vi "_PC_Pub_ExpCondi getAttributeValue.vi"(7 "attrName":string="Script", 8 "error in (no error)":errorcluster, 11 "expCondiVariant":variant) -> (0 "error out":errorcluster, 3 "attrValue":cluster{"Label":string, "Value":variant})   [LabVIEW 2018]
uses:
  <vilib>/Utility/error.llb/Error Cluster From Error Code.vi
  <vilib>/ErrorRing/Error Ring.xnode
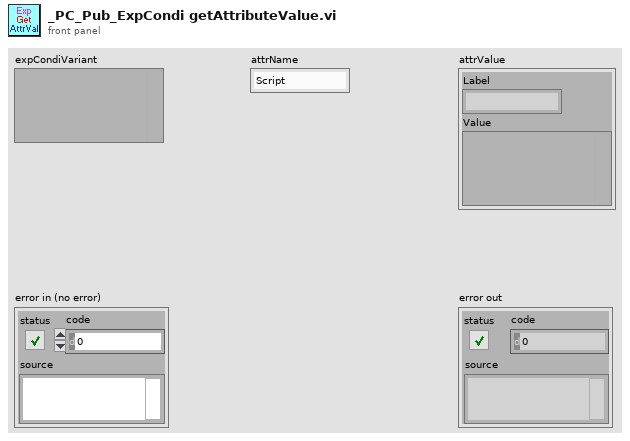
[diagram p1: front panel]
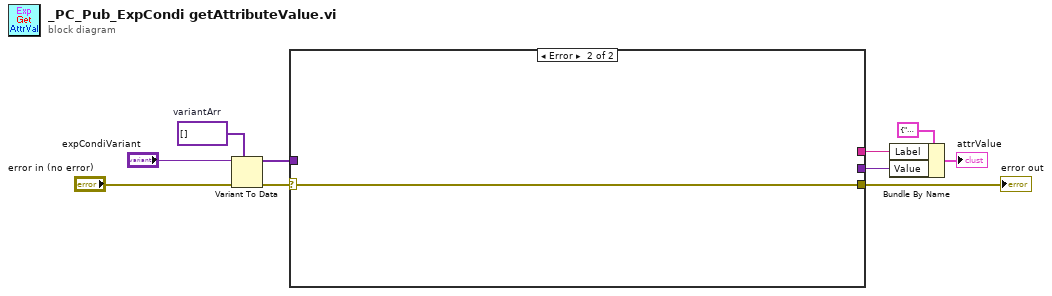
[diagram p0: block diagram]
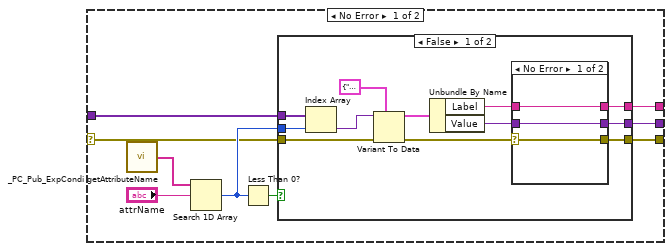
[diagram p2: hidden frame]
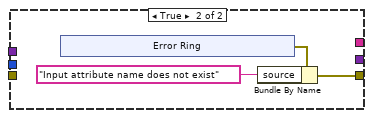
[diagram p4: hidden frame]
diagram:
  w8 = variant[] []  # variantArr
  n1 = Variant To Data(error in="error in (no error)", type=w8, Variant="expCondiVariant") -> (data=w7:variant[], error out=w6:errorcluster)
  n2 = case shown="Error" w6 {
    selector: w6 -> [w13 w43]
    tunnel: [w17 w43] -> w10
    tunnel: w7 -> [w16 _]
    tunnel: [w12 _] -> w4
    tunnel: [w11 _] -> w3
    frame No Error {
      n3 = call "_PC_Pub_ExpCondi getAttributeName.vi"() -> ("attrName"=w19:string[])
      n4 = Search 1D Array(1D array=w19, element="attrName") -> (index of element=w15:i32)  [unwired: 1 in]
      n5 = Less Than 0?(x=w15) -> (x < 0?=w18:bool)
      n6 = case shown="False" w18 {
        tunnel: [w24 w36] -> w17
        tunnel: w16 -> [w31 _]
        tunnel: w15 -> [w30 _]
        tunnel: w13 -> [w26 _]
        tunnel: [w21 _] -> w12
        tunnel: [w20 _] -> w11
        frame False {
          n7 = Index Array(array=w31, index=w30) -> (element=w29:variant)
          n8 = Variant To Data(error in=w26, type=cluster{"Label":string, "Value":variant} {"Label"="", "Value"=variant} ("element"), Variant=w29) -> (data=w27:cluster{"Label":string, "Value":variant}, error out=w25:errorcluster)
          n9 = Unbundle By Name(w27) -> ("Label"=w23:string, "Value"=w22:variant)
          n10 = case shown="No Error" w25 {
            selector: w25 -> [w34 w35]
            tunnel: [w34 w35] -> w24
            tunnel: w23 -> [w33 _]
            tunnel: w22 -> [w32 _]
            tunnel: [w33 _] -> w21
            tunnel: [w32 _] -> w20
            frame No Error {
            }
            frame Error {
            }
          }
        }
        frame True {
          n11 = xnode "Error Ring"() -> ("error out"=w38:errorcluster)
          n12 = Bundle By Name(cluster=w38, "source"="Input attribute name does not exist") -> (w36:errorcluster)
        }
      }
    }
    frame Error {
    }
  }
  "error out" <- w10
  n13 = Bundle By Name(cluster=cluster{"Label":string, "Value":variant} {"Label"="", "Value"=variant} ("element"), "Label"=w4, "Value"=w3) -> (→"attrValue":cluster{"Label":string, "Value":variant})
